vi "扇形面积.vi"(8 "Angle（n）":dbl, 11 "Radious":dbl) -> (3 "Area":dbl=nan)   [LabVIEW 2011]
doc: "功能：\n计算给定圆心角和半径构成的扇形面积。\n\n计算公式：\nA=n*Pi*r^2/360,其中n为圆心角，单位为度，r为半径。"
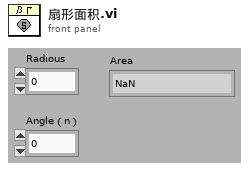
[diagram p1: front panel]
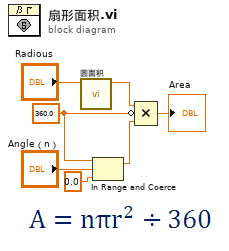
[diagram p0: block diagram]
diagram:
  w2 = 360.0 ("上限")
  n1 = call "圆面积.vi"("Radious"="Radious") -> ("Area"=w5:dbl)  [unwired: 10 in]
  n2 = In Range and Coerce(upper limit=w2, x="Angle（n）", lower limit=0.0 ("下限")) -> (coerced(x)=w1:dbl)  [unwired: 1 out]
  n3 = Compound Arithmetic op=MULTIPLY(w5, invert w2, w1) -> (→"Area":dbl)
